vi "AlliGator Get Phasor Harmonic Components.vi"(11 "Stored Phasor Harmonics":T1[](array[typedef])) -> (0 "Phasor Harmonic Orders":u8[](array[numeric]), 1 "Phasor Harmonic Base Fequencies":dbl[unit][](array[numeric]), 2 "Phasor Harmonic Frequencies":dbl[unit][](array[numeric]), 3 "Phasor Harmonic Names":string[](array[string]), 4 "Phasor Harmonic Parameter Strings":string[](array[string]), 5 "Phasor Harmonic Dataset File Paths":path[](array[path]), 6 "Phasor Harmonic Checksums":u64[](array[numeric]))   [LabVIEW 2021]
uses:
  Phasor/Phasor Harmonic Data.ctl
  Phasor/Phasor.lvlib
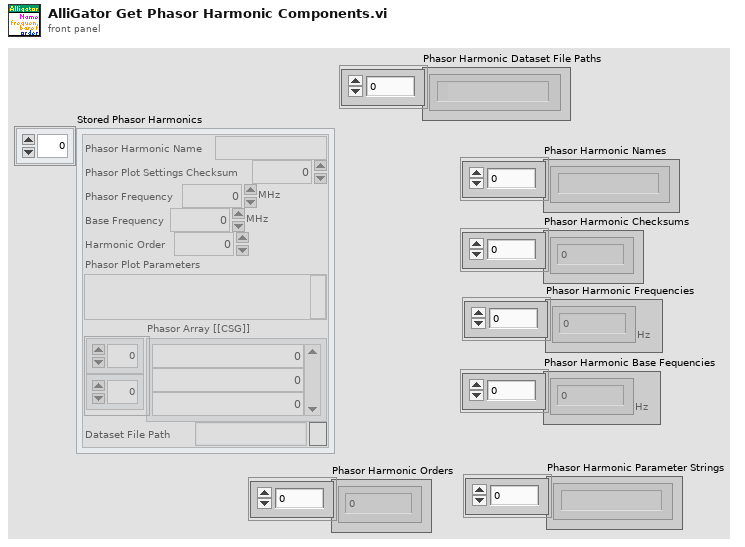
[diagram p1: front panel]
types:
  T1 = typedef "Phasor.lvlib/Phasor Harmonic Data.ctl" = cluster{"Phasor Harmonic Name":string, "Phasor Plot Settings Checksum":u64, "Phasor Frequency":dbl[unit], "Base Frequency":dbl[unit], "Harmonic Order":u8, "Phasor Plot Parameters":string, "Phasor Array [[CSG]]":csg[][], "Dataset File Path":path}
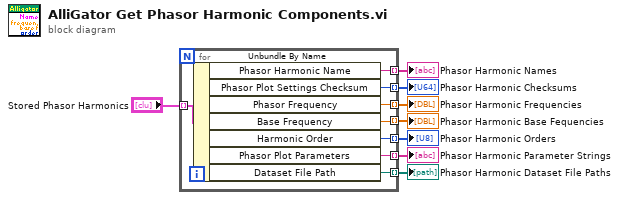
[diagram p0: block diagram]
diagram:
  n1 = for {
    tunnel: "Stored Phasor Harmonics" -> [w16] mode=indexing
    tunnel: [w15] -> w6 mode=indexing
    tunnel: [w14] -> w7 mode=indexing
    tunnel: [w13] -> w5 mode=indexing
    tunnel: [w12] -> w4 mode=indexing
    tunnel: [w11] -> w3 mode=indexing
    tunnel: [w10] -> w2 mode=indexing
    tunnel: [w9] -> w1 mode=indexing
    n2 = Unbundle By Name(w16) -> ("Phasor Harmonic Name"=w14:string, "Phasor Plot Settings Checksum"=w15:u64, "Phasor Frequency"=w13:dbl[unit], "Base Frequency"=w12:dbl[unit], "Harmonic Order"=w11:u8, "Phasor Plot Parameters"=w10:string, "Dataset File Path"=w9:path)
  }
  "Phasor Harmonic Names" <- w7
  "Phasor Harmonic Checksums" <- w6
  "Phasor Harmonic Frequencies" <- w5
  "Phasor Harmonic Base Fequencies" <- w4
  "Phasor Harmonic Orders" <- w3
  "Phasor Harmonic Parameter Strings" <- w2
  "Phasor Harmonic Dataset File Paths" <- w1
